vi "DaxInternaMultiTrig.vi"(1 "Motion Settings":T1={"No Motion?"=FALSE, "Motion System"=enum."NI 735x", "Motion Bd ID"=1, "Motion Profile"="SMAC1", "# Axis"=1, "Reverse Z axis?"=TRUE, "SMAC Axis"=0, "scan pair"=enum."y-(x) scan", "RT fps"=6.0, "Steps per mm"=[1000, 1000, 1000, 1000], "Motor Parameters"={"velocity ct/s"=[10000.0, 10000.0, 10000.0, 50000.0], "accel ct/s^2"=[50000.0, 50000.0, 50000.0, 200000.0]}, "One Way Scan"=FALSE, "Reverse One Way Scan"=FALSE, "Global Position (mm)"=[], "Plane"=0, "Distance between\nscan lines (um)"=0.0, "Distance between\nscan planes (um)"=0.0, "number of scan planes"=1, "Total steps in line"=0, "Xtra plane\ndistance  (um)"=100, "Xtra planes "=1, "Add Axis"=FALSE, "overshoot cts"=200, "BKPT Shift"=0, "Scan Start Time (ms)"=0, "ESP VISA"="GPIB::1::INSTR", "3rd Axis"=1, "GL Ref Out"=refnum, "Galil Address"=""} {"3rd Axis" items=["x", "y", "z", "w"]; "Xtra planes" min=1; "Xtra plane\ndistance  (um)" min=0; "Distance between\nscan planes (um)" format="%.2f"; "Distance between\nscan lines (um)" format="%.2f"; "SMAC Axis" items=["None"=0, "Axis 1"=1, "Axis 2"=2, "Axis 3"=3, "Axis 4"=4, "Axis 5"=5, "Axis 6"=6, "Axis 7"=7, "Axis 8"=8, "Vector Space 1"=17, "Vector Space 2"=18, "Vector Space 3"=19, "Vector Space 4"=20]; "Motion Bd ID" min=1 max=32 step=1}, 5 "Digitizer Settings":T5={"Digitizer delay (us) "=0.0, "rf points per line"=2048, "lines per plane"=128, "Samp Rate (Hz)"=100000000.0, "Additional dig delay (us)"=0.0, "Voltage Scale"=0.4, "Pre-Looks"=0, "Offset delay (us)"=0.0, "bits A/D"=8, "Avg Num"=1, "DigTimeOut"=5.0, "Rel Dig Delay"=0.0, "Dig Ch"=0, "LeCroyCluster"={"LeCroy Channels"=[TRUE, FALSE, FALSE, FALSE], "LC read pt offset"=0.0, "Sweep Avg"=FALSE}, "Main Digitizer"=enum."NI Digitizer", "Dig Config"=enum."Single channel", "Digitizer ID Cluster"={"Acqiris/Alazar/SP ID"=[], "NI Instr Handles"=[], "LeCroy VISA"="", "GaGe Handle"={"Handle"=0, "Sample size"=0, "Resolution"=0, "Offset"=0, "Channels"=0, "Boards"=0}, "ATS Ref"="ATS9350", "Acqiris Address"=["PCI::INSTR0"], "ADQRef"=refnum, "adq_cu_ptr"=refnum}, "Trigger Settings"={"Trig Source"=1, "Trig Coupling"=0, "Trig Slope"=0, "Level (mV)"=1500.0}, "Bulk Acq"=FALSE, "Bulk Start Indexes"=[], "Data Ref RF"=refnum, "NI ID/Channel"=[], "Total Dig CH"=1, "Xtra Ann Trig delay (us)"=10.0, "Fix Z Delay?"=FALSE, "One Way Transmission?"=FALSE, "Data Ref Log"=refnum} {"Trigger Settings"."Trig Slope" items=["Positive", "Negative"]; "Trigger Settings"."Level (mV)" format="%.2f"; "Trigger Settings"."Trig Coupling" items=["DC 1 MOhm", "AC 1 MOhm", "DC 50 Ohm", "AC 50 Ohm"]; "Trigger Settings"."Trig Source" items=["Chan 1", "External"]; "Rel Dig Delay" format="%.2f"; "DigTimeOut" format="%.2f"; "Avg Num" min=1; "Offset delay (us)" format="%.2f"; "Additional dig delay (us)" format="%.2f"; "Digitizer delay (us)" format="%.2f"}, 6 "XMIT":bool[](array[boolean])=[TRUE, TRUE, TRUE, TRUE, TRUE], 7 "extra time":dbl=1e-06 format="%^.2e", 8 "Axis":u16(ring)=1 caption="Axis or Vector Space" items=["Axis 1"=1, "Axis 2"=2, "Axis 3"=3, "Axis 4"=4, "Axis 5"=5, "Axis 6"=6, "Axis 7"=7, "Axis 8"=8, "Vector Space 1"=17, "Vector Space 2"=18, "Vector Space 3"=19, "Vector Space 4"=20], 10 "error in":errorcluster) -> (3 "error out":errorcluster)   [LabVIEW 2022 SP3]
uses:
  Digitizers/-DigitizerRoutines/DigitizerSettings.ctl
  Digitizers/-DigitizerRoutines/Digitizer.ctl
  Digitizers/-DigitizerRoutines/DigConfig.ctl
  Digitizers/-DigitizerRoutines/DigitizerID.ctl
  C:/Windows/System32/ADQAPI_dotNet_helper.dll
  Motion Controllers/NI_controller/-NI_MotionRoutines/MotionParameters.ctl
  Motion Controllers/NI_controller/-NI_MotionRoutines/MotionSys.ctl
  Motion Controllers/-MotionRoutines/ScanAxis.ctl
  Motion Controllers/-MotionRoutines/3rdAxis.ctl
  Switch Modules/SwitchGlobals.vi
  PulserGlobals.vi
panel:
  out "Array":dbl[](array[numeric]) format="%#_3e"
  # "Counter 1 output is the BNC on grey box."
  # "Trigger source comes from Gate of CTR0 (PFI9)\n\nThe NI trigger connector routes to CTR0 Gate"
  # "1-D and 2-D B scan settings"
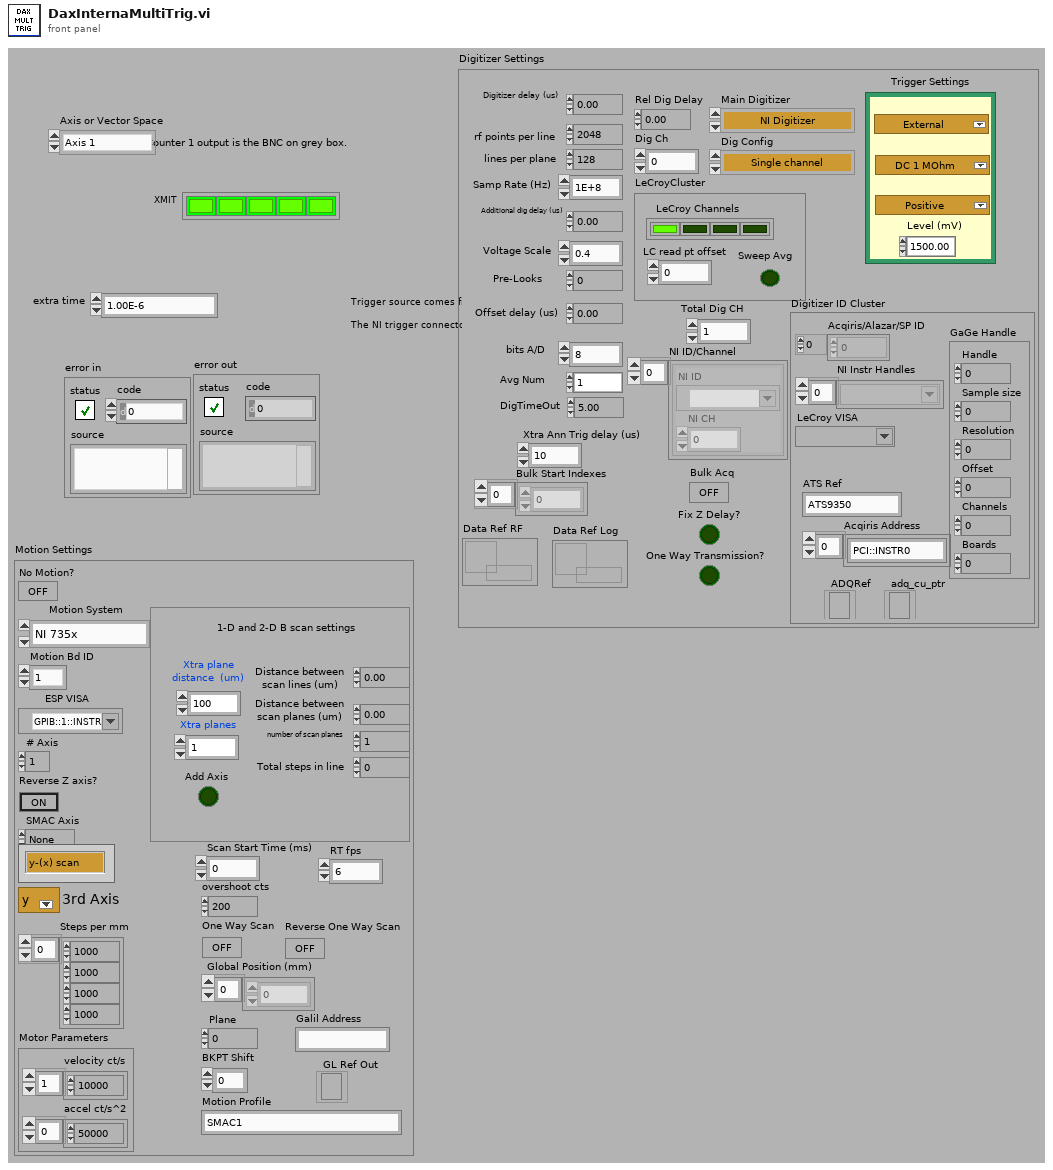
[diagram p1: front panel]
types:
  T1 = typedef "MotionParameters.ctl" = cluster{"No Motion?":bool, "Motion System":T2, "Motion Bd ID":u8, "Motion Profile":string, "# Axis":i8, "Reverse Z axis?":bool, "SMAC Axis":u16, "scan pair":T3, "RT fps":sgl, "Steps per mm":i32[], "Motor Parameters":cluster{"velocity ct/s":dbl[], "accel ct/s^2":dbl[]}, "One Way Scan":bool, "Reverse One Way Scan":bool, "Global Position (mm)":dbl[], "Plane":i32, "Distance between\nscan lines (um)":sgl, "Distance between\nscan planes (um)":sgl, "number of scan planes":i32, "Total steps in line":i32, "Xtra plane\ndistance  (um)":i32, "Xtra planes ":i32, "Add Axis":bool, "overshoot cts":i32, "BKPT Shift":i32, "Scan Start Time (ms)":u32, "ESP VISA":refnum<visa-resource-name>, "3rd Axis":T4, "GL Ref Out":refnum<k7>, "Galil Address":string}
  T2 = typedef "MotionSys.ctl" = enum16{"MM3000", "NI 735x", "Newport ESP", "No Motion Card", "Galil"}
  T3 = typedef "ScanAxis.ctl" = enum16{"y-(x) scan", "x-(y) scan", "z-(x) scan", "z-(y) scan", "y-(z) scan", "x-(z) scan", "w-(x) scan", "w-(y) scan", "w-(z) scan", "x-(w) scan", "y-(w) scan", "z-(w) scan"}
  T4 = typedef "3rdAxis.ctl" = u16
  T5 = typedef "DigitizerSettings.ctl" = cluster{"Digitizer delay (us) ":dbl, "rf points per line":i32, "lines per plane":i32, "Samp Rate (Hz)":dbl, "Additional dig delay (us)":dbl, "Voltage Scale":dbl, "Pre-Looks":i32, "Offset delay (us)":dbl, "bits A/D":i8, "Avg Num":i32, "DigTimeOut":sgl, "Rel Dig Delay":sgl, "Dig Ch":i32, "LeCroyCluster":cluster{"LeCroy Channels":bool[], "LC read pt offset":dbl, "Sweep Avg":bool}, "Main Digitizer":T6, "Dig Config":T7, "Digitizer ID Cluster":T8, "Trigger Settings":cluster{"Trig Source":u16, "Trig Coupling":u16, "Trig Slope":u16, "Level (mV)":dbl}, "Bulk Acq":bool, "Bulk Start Indexes":i32[], "Data Ref RF":refnum<data-value>, "NI ID/Channel":cluster{"NI ID":refnum<k15>, "NI CH":i32}[], "Total Dig CH":i32, "Xtra Ann Trig delay (us)":dbl, "Fix Z Delay?":bool, "One Way Transmission?":bool, "Data Ref Log":refnum<data-value>}
  T6 = typedef "Digitizer.ctl" = enum16{"Acqiris Digitizer", "NI Digitizer", "LeCroy", "GaGe", "AlazarTech", "No Digitizer", "Teledyne"}
  T7 = typedef "DigConfig.ctl" = enum16{"Single channel", "2 Chans w/ 2 Acqiris", "2 Chans w/ 1 Acqiris", "5-CH Pulser New", "5-CH pulser w/ ann array", "5-pass style ann array", "Empty"}
  T8 = typedef "DigitizerID.ctl" = cluster{"Acqiris/Alazar/SP ID":u32[], "NI Instr Handles":refnum<k15>[], "LeCroy VISA":refnum<visa-resource-name>, "GaGe Handle":cluster{"Handle":u32, "Sample size":u32, "Resolution":i32, "Offset":i32, "Channels":u32, "Boards":u32}, "ATS Ref":string, "Acqiris Address":string[], "ADQRef":refnum<k24>, "adq_cu_ptr":refnum<k24>}
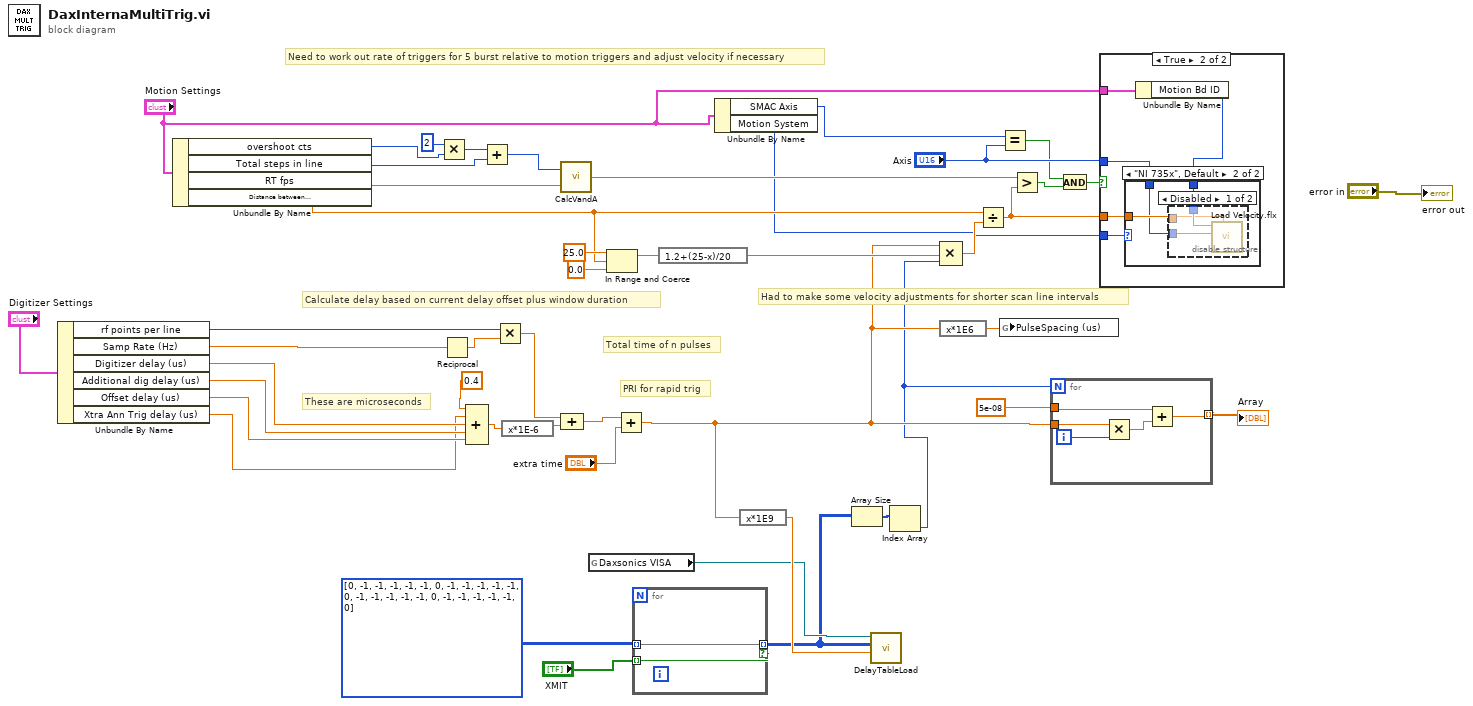
[diagram p0: block diagram]
diagram:
  # "PRI for rapid trig"
  # "Had to make some velocity adjustments for shorter scan line intervals"
  # "Total time of n pulses"
  # "Need to work out rate of triggers for 5 burst relative to motion triggers and adjust velocity if necessary"
  # "Calculate delay based on current delay offset plus window duration"
  # "These are microseconds"
  n1 = Unbundle By Name("Digitizer Settings") -> ("rf points per line"=w24:i32, "Samp Rate (Hz)"=w23:dbl, "Digitizer delay (us)"=w22:dbl, "Additional dig delay (us)"=w21:dbl, "Offset delay (us)"=w20:dbl, "Xtra Ann Trig delay (us)"=w11:dbl)
  n2 = Unbundle By Name("Motion Settings") -> ("overshoot cts"=w18:i32, "Total steps in line"=w17:i32, "RT fps"=w16:sgl, "Distance between\nscan lines (um)"=w15:sgl)
  n3 = Multiply(x=2, y=w18) -> (x*y=w44:i32)
  n4 = Reciprocal(x=w23) -> (1/x=w46:dbl)
  n5 = Compound Arithmetic op=ADD(0.4 ("y"), w11, w22, w21, w20) -> (w33:dbl)
  n6 = Add(x=w44, y=w17) -> (x+y=w43:i32)
  n7 = Multiply(x=w24, y=w46) -> (x*y=w47:dbl)
  n8 = expression code="x*1E-6"(w33) -> (w32:dbl)
  n9 = call "CalcVandA.vi"("distance"=w43, "fps"=w16) -> ("Velocity"=w42:dbl)  [unwired: 2 out]
  n10 = Compound Arithmetic op=ADD(w47, w32) -> (w40:dbl)
  n11 = global read "PulserGlobals.vi" "Daxsonics VISA"() -> (w5:refnum<visa-resource-name>)
  n12 = In Range and Coerce(upper limit=sgl 25.0, x=w15, lower limit=sgl 0.0) -> (coerced(x)=w39:sgl)  [unwired: 1 out]
  n13 = Add(x=w40, y="extra time") -> (x+y=w9:dbl)
  n14 = for {
    tunnel: i32[][] [[0, -1, -1, -1, -1], [-1, 0, -1, -1, -1], [-1, -1, 0, -1, -1], [-1, -1, -1, 0, -1], [-1, -1, -1, -1, 0]] ("Delay Table (ns)") -> [w49] mode=indexing
    tunnel: [w49] -> w4 mode=indexing if=w48
    tunnel: "XMIT" -> [w48] mode=indexing
  }
  n15 = expression code="1.2+(25-x)/20"(w39) -> (w36:sgl)
  n16 = Unbundle By Name("Motion Settings") -> ("SMAC Axis"=w14:u16, "Motion System"=w13:T2)
  n17 = expression code="x*1E9"(w9) -> (w6:dbl)
  n18 = Array Size(array=w4) -> (size(s)=w3:i32[])
  n19 = call "DelayTableLoad.vi"("PRI (ns)"=w6, "Delay Table (ns)"=w4, "VISA Refnum in"=w5) -> ()  [unwired: 9 in]
  n20 = Index Array(array=w3) -> (element=w1:i32)  [unwired: 1 in]
  n21 = Compound Arithmetic op=MULTIPLY(w9, w36, w1) -> (w35:dbl)
  n22 = expression code="x*1E6"(w9) -> (w12:dbl)
  n23 = Divide(x=w15, y=w35) -> (x/y=w41:dbl)
  n24 = Equal?(x=w14, y="Axis") -> (x = y?=w27:bool)
  n25 = global write "SwitchGlobals.vi" "PulseSpacing (us)"(w12) -> ()
  n26 = Greater?(x=w42, y=w41) -> (0:w29:bool)
  n27 = for {
    N: w1 -> [_]
    tunnel: w9 -> [w54]
    tunnel: 5e-08 ("x") -> [w52]
    tunnel: [w50] -> w26 mode=indexing
    i -> [w51]
    n28 = Multiply(x=w54, y=w51) -> (x*y=w53:dbl)
    n29 = Add(x=w52, y=w53) -> (x+y=w50:dbl)
  }
  "Array" <- w26
  n30 = And(x=w27, y=w29) -> (x .and. y?=w28:bool)
  n31 = case shown="True" w28 {
    tunnel: w41 -> [_ w59]
    tunnel: "Axis" -> [_ w58]
    tunnel: w13 -> [_ w57]
    tunnel: "Motion Settings" -> [_ w56]
    frame False {
    }
    frame True {
      n32 = Unbundle By Name(w56) -> ("Motion Bd ID"=w55:u8)
      n33 = case shown="\"NI 735x\", Default" w57 {
        tunnel: w55 -> [_ w62]
        tunnel: w59 -> [_ w61]
        tunnel: w58 -> [_ w60]
        frame "No Motion Card" {
        }
        frame "NI 735x", Default {
          n34 = disable-structure shown="Disabled" {
            disable-tunnel: w62 -> [w65 _]
            disable-tunnel: w61 -> [w64 _]
            disable-tunnel: w60 -> [w63 _]
            frame Disabled {
              n35 = call <vilib>:"Load Velocity.flx"("Velocity (10000)"=w64, "Axis or Vector Space"=w63, "Board ID"=w65) -> ()  [unwired: 1 in, 6 out]
            }
            frame Enabled {
            }
          }
        }
      }
    }
  }
  "error out" <- "error in"
